vi "ReadFromFIFO.vi"() -> (2 "This is what I told you!":string)   [LabVIEW 2011]
doc: "Elizabeth Mahon\nNot finished yet\nBased off of example from LabView and IGVC 3.2.1 Read VectorNav.\n\nDoesn't take in anything, gives string result.\n\nNot sure what folder this should be in..."
uses:
  <vilib>/rvi/interface/nirviOpenFPGA/nirviOpenFPGA.xnode
  WriteToFIFO.vi
  <vilib>/rvi/interface/nirviMethod/nirviMethod.xnode
  <vilib>/FPGAPlugInAG/Dynamic/niLvFpga_ReadFifo_Dynamic.vi
  <vilib>/rvi/errors/niLvFpgaMergeErrorWithErrorCode.vi
  2-RIO/2 Globals/2 Global.vi
panel:
  in  "Status":enum16{"Waiting", "Reading", "Time Out!"}(ring)
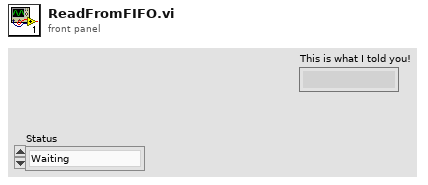
[diagram p1: front panel]
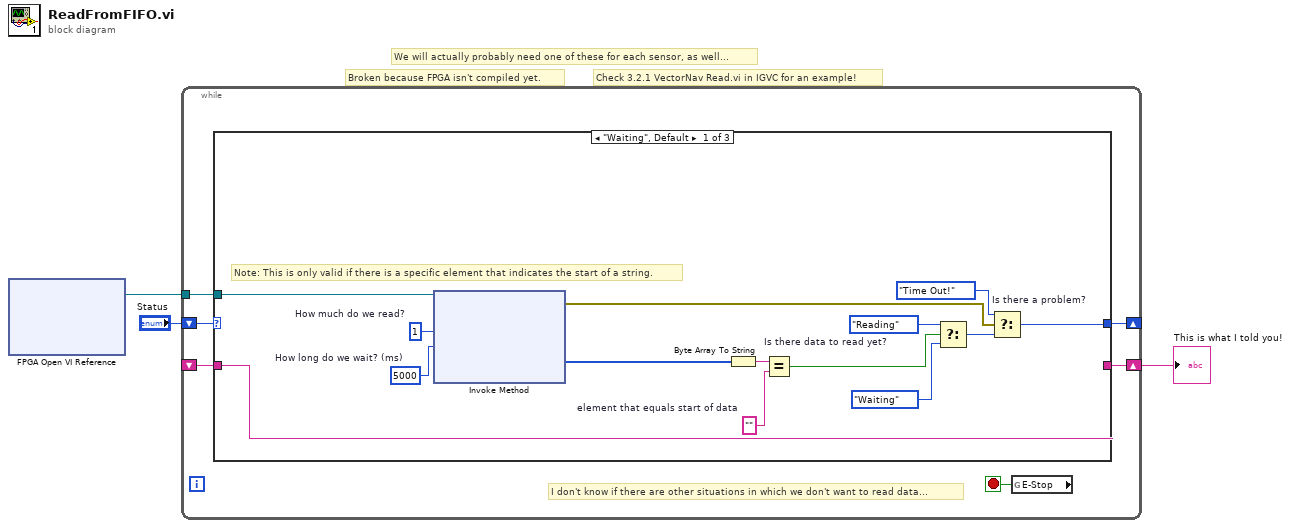
[diagram p0: block diagram]
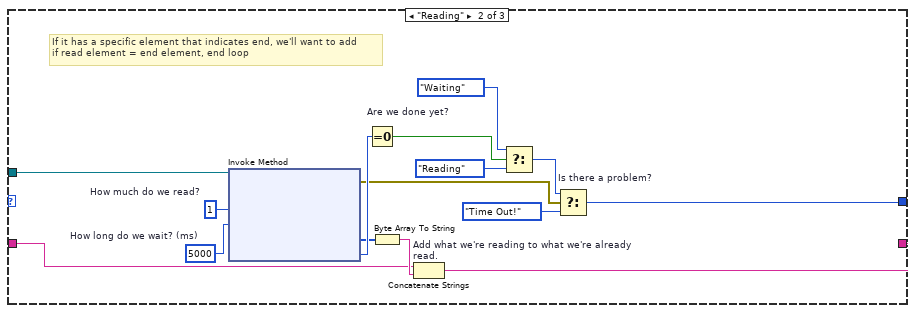
[diagram p2: hidden frame]
diagram:
  # "Broken because FPGA isn't compiled yet."
  # "Check 3.2.1 VectorNav Read.vi in IGVC for an example!"
  # "We will actually probably need one of these for each sensor, as well..."
  n1 = xnode "FPGA Open VI Reference"() -> ("FPGA VI Reference Out"=w3:refnum<k20>)  [unwired: 2 in, 1 out]
  n2 = while {
    tunnel: w3 -> [w9]
    shift-right: [w7] -> w2
    shift-left: _ -> [w8]
    shift-right: [w6] -> _
    shift-left: "Status" -> [w5]
    stop <- w4 stop-if-true
    # "I don't know if there are other situations in which we don't want to read data..."
    n3 = case shown="\"Waiting\", Default" w5 {
      selector: w5 -> [_ _ w40]
      tunnel: w9 -> [w21 w38 _]
      tunnel: w8 -> [w20 w32 w39]
      tunnel: [w20 w31 w39] -> w7
      tunnel: [w10 w24 w40] -> w6
      frame "Waiting", Default {
        w17 = ""  # element that equals start of data
        w22 = 5000  # How long do we wait? (ms)
        w23 = u32 1  # How much do we read?
        # "Note: This is only valid if there is a specific element that indicates the start of a string."
        n4 = xnode "Invoke Method"("FPGA VI Reference In"=w21, "Number of Elements"=w23, "Timeout (ms)"=w22) -> ("error out"=w13:errorcluster, "Data"=w19:i16[])  [unwired: 1 in, 2 out]
        n5 = Byte Array To String(unsigned byte array=w19) -> (string=w18:string)
        n6 = Equal? "Is there data to read yet?"(x=w18, y=w17) -> (x = y?=w16:bool)
        n7 = Select(t=enum16{"Waiting", "Reading", "Time Out!"}."Reading" ("Status"), s=w16, f=enum16{"Waiting", "Reading", "Time Out!"}."Waiting" ("Status")) -> (s? t:f=w12:enum16{"Waiting", "Reading", "Time Out!"})
        n8 = Select "Is there a problem?"(t=enum16{"Waiting", "Reading", "Time Out!"}."Time Out!", s=w13, f=w12) -> (s? t:f=w10:enum16{"Waiting", "Reading", "Time Out!"})
      }
      frame "Reading" {
        w36 = 5000  # How long do we wait? (ms)
        w37 = u32 1  # How much do we read?
        # "If it has a specific element that indicates end, we'll want to add\nif read element = end element, end loop"
        n9 = xnode "Invoke Method"("FPGA VI Reference In"=w38, "Number of Elements"=w37, "Timeout (ms)"=w36) -> ("error out"=w27:errorcluster, "Data"=w34:i16[], "Elements Remaining"=w35:u32)  [unwired: 1 in, 1 out]
        n10 = Equal To 0? "Are we done yet?"(x=w35) -> (x = 0?=w28:bool)
        n11 = Byte Array To String(unsigned byte array=w34) -> (string=w33:string)
        n12 = Concatenate Strings "Add what we're reading to what we're already read."(w32, w33) -> (w31:string)
        n13 = Select(t=enum16{"Waiting", "Reading", "Time Out!"}."Waiting" ("Status"), s=w28, f=enum16{"Waiting", "Reading", "Time Out!"}."Reading" ("Status")) -> (s? t:f=w25:enum16{"Waiting", "Reading", "Time Out!"})
        n14 = Select "Is there a problem?"(t=w25, s=w27, f=enum16{"Waiting", "Reading", "Time Out!"}."Time Out!") -> (s? t:f=w24:enum16{"Waiting", "Reading", "Time Out!"})
      }
      frame "Time Out!" {
        # "error or something. Not sure what to do."
      }
    }
    n15 = global read "2 Global.vi" "E-Stop"() -> (w4:bool)
  }
  "This is what I told you!" <- w2
